vi "ClsSaveConfig.vi"(8 "error in (no error)":errorcluster, 11 "ClsConfigureValues":T1) -> (0 "error out":errorcluster)   [LabVIEW 2015]
uses:
  TypeDefs/ClsConfigureValues.ctl
  <vilib>/Utility/xml.llb/Write to XML File(string).vi
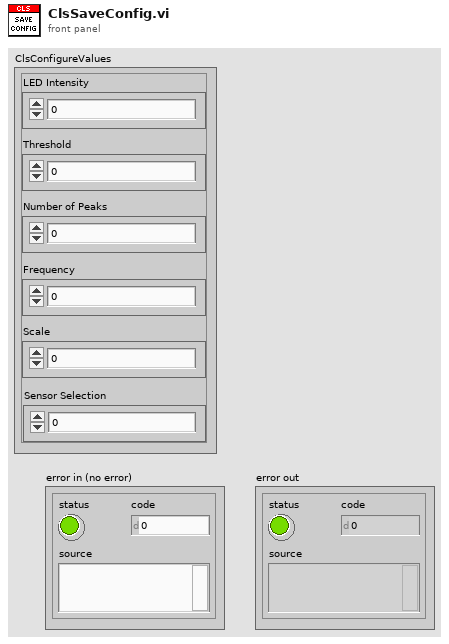
[diagram p1: front panel]
types:
  T1 = typedef "ClsConfigureValues.ctl" = cluster{"LED Intensity":dbl, "Threshold":dbl, "Number of Peaks":dbl, "Frequency":dbl, "Scale":dbl, "Sensor Selection":dbl}
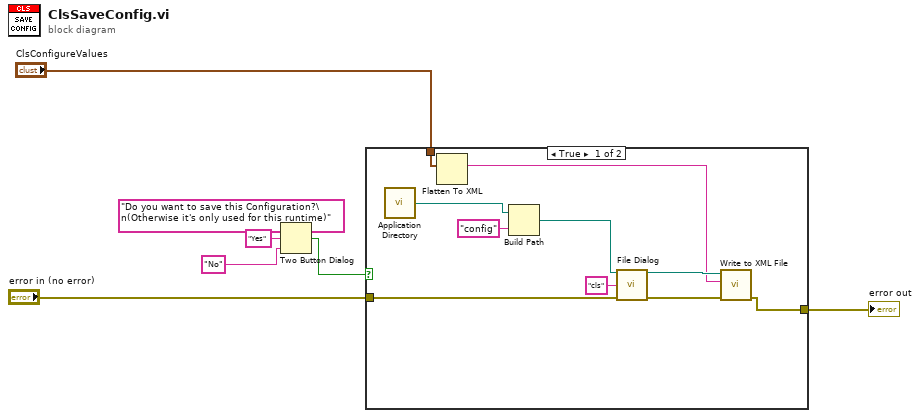
[diagram p0: block diagram]
diagram:
  n1 = Two Button Dialog(message="Do you want to save this Configuration?\n(Otherwise it's only used for this runtime)", 1:"No" ("F button name (\"Cancel\")"), 2:"Yes" ("T button name (\"OK\")")) -> (T button?=w2:bool)
  n2 = case shown="True" w2 {
    tunnel: "error in (no error)" -> [w17 w18]
    tunnel: [w8 w18] -> w4
    tunnel: "ClsConfigureValues" -> [w12 _]
    frame True {
      n3 = call <vilib>:"Application Directory.vi"() -> ("Application Directory"=w16:path)
      n4 = Flatten To XML(anything=w12) -> (xml string=w10:string)
      n5 = Build Path(base path=w16, name or relative path="config") -> (appended path=w14:path)
      n6 = call "File Dialog"("start path"=w14, "default name"="cls", "error in"=w17) -> ("selected path"=w11:path, "error out"=w9:errorcluster)  [unwired: 9 in, 2 out]
      n7 = call-poly <vilib>:"Write to XML File.vi"("error in (no error)"=w9, "XML Input"=w10, "XML File Path"=w11) -> ("error out"=w8:errorcluster)  [unwired: 6 in, 2 out]
    }
    frame False {
    }
  }
  "error out" <- w4
